vi "GoalOrNot.vi"(8 "goal x":dbl, 9 "goal width":dbl, 10 "ball x":dbl, 11 "ball y":dbl) -> (3 "Goal or Not":bool)   [LabVIEW 2017]
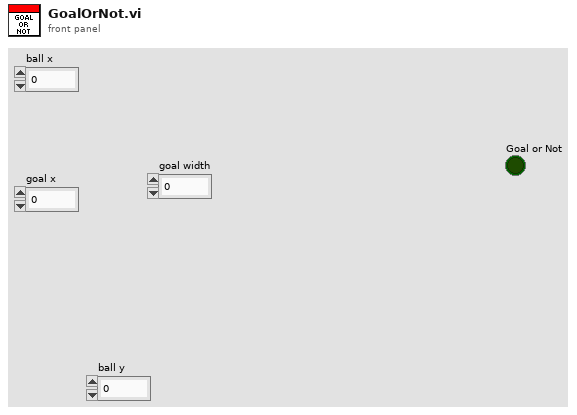
[diagram p1: front panel]
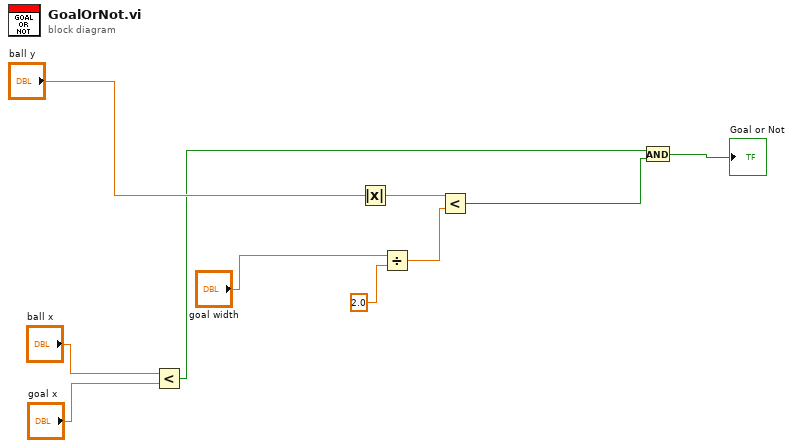
[diagram p0: block diagram]
diagram:
  n1 = Less?(x="ball x", y="goal x") -> (x < y?=w1:bool)
  n2 = Absolute Value(x="ball y") -> (abs(x)=w9:dbl)
  n3 = Divide(x="goal width", y=2.0) -> (x/y=w5:dbl)
  n4 = Less?(x=w9, y=w5) -> (x < y?=w8:bool)
  n5 = And(x=w1, y=w8) -> (x .and. y?=→"Goal or Not":bool)
